vi "Set SA Path.vi"(0 "SA Path in":refnum<class "SA 18GHz Path.lvclass">, 11 "error in":errorcluster) -> (4 "SA Path out":refnum<class "SA 18GHz Path.lvclass">, 15 "error out":errorcluster)   [LabVIEW 2023, in "RFFixtureCharact.RFPM.lvlib" / "SA 18GHz Path.lvclass"]
uses:
  SA 18GHz Path.lvclass
  C:/srd-semi-rfcal-software/AuxTools/STSRFFixtureCharactUtility/Source/Code Modules/Common/Base Classes/Path/Path.lvclass
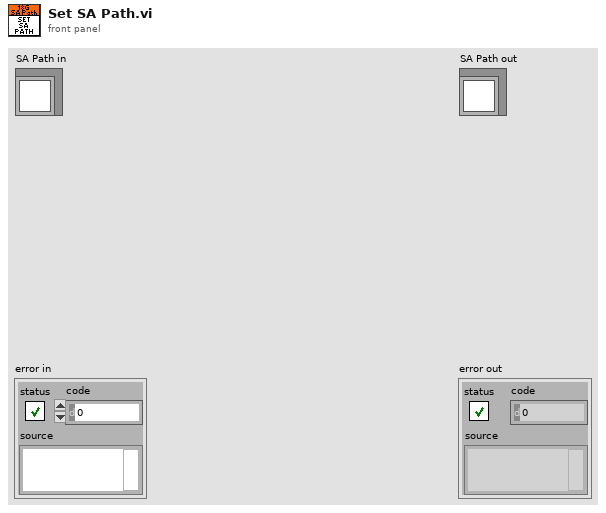
[diagram p1: front panel]
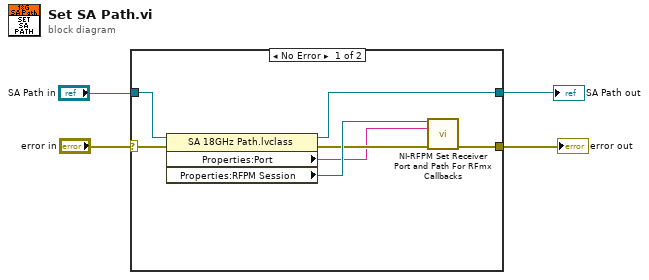
[diagram p0: block diagram]
diagram:
  n1 = case shown="No Error" "error in" {
    selector: "error in" -> [w10 w12]
    tunnel: [w6 w13] -> w2
    tunnel: "SA Path in" -> [w11 w13]
    tunnel: [w7 w12] -> w1
    frame No Error {
      n2 = property class="SA 18GHz Path.lvclass"(reference=w11, error in=w10) -> (reference out=w6:refnum<class "SA 18GHz Path.lvclass">, error out=w8:errorcluster, "Properties:Port"=w5:string, "Properties:RFPM Session"=w9:refnum<k15>)
      n3 = call <instrlib>:"NI-RFPM Set Receiver Port and Path For RFmx Callbacks.vi"("instrument handle"=w9, "Port"=w5, "error in"=w8) -> ("error out"=w7:errorcluster)  [unwired: 11 in, 1 out]
    }
    frame Error {
    }
  }
  "error out" <- w1
  "SA Path out" <- w2
